vi "Modbus FVIR Boolean Decode.vi"(8 "error in":errorcluster, 10 "Input Registers":u16[](array[numeric]), 11 "PLC Data":T1) -> (0 "error out":errorcluster, 3 "PLC Data Out":T1)   [LabVIEW 2020, in "Modbus.lvlib"]
uses:
  Modbus.lvlib
  Modbus PLC Data All.ctl
  Modbus FVIR Control.ctl
  Modbus LDO Control.ctl
  WritingDataFile/Data to Save.ctl
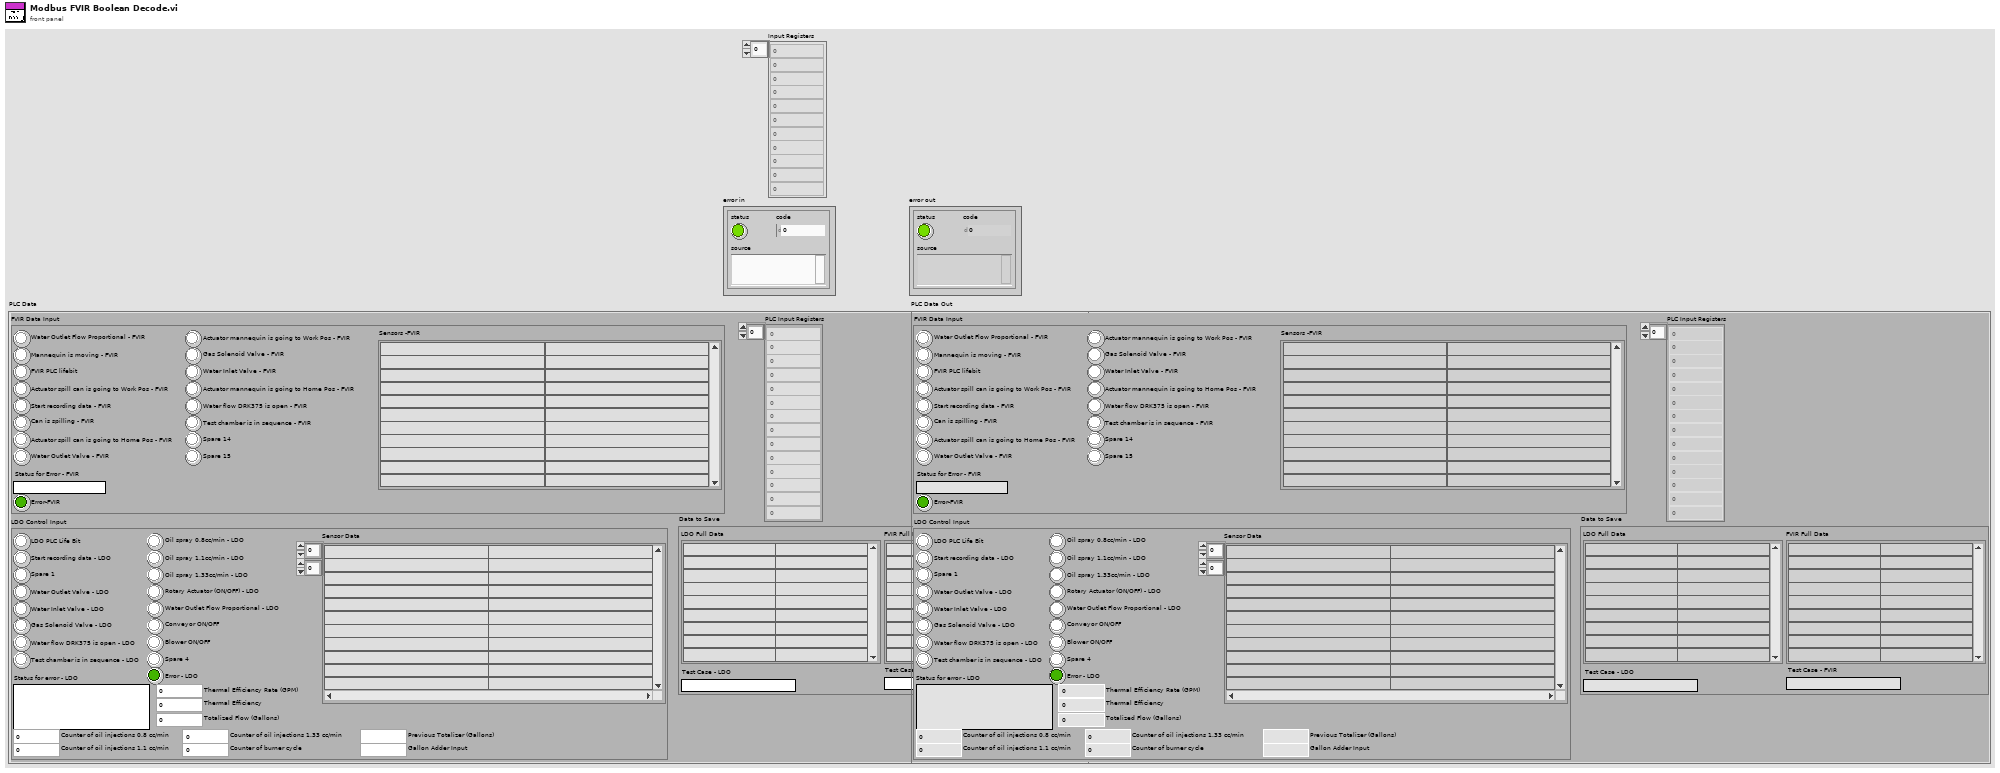
[diagram p1: front panel]
types:
  T1 = typedef "Modbus PLC Data All.ctl" = cluster{"FVIR Data Input":T2, "LDO Control Input":T3, "PLC Input Registers":i16[], "Data to Save":T4}
  T2 = typedef "Modbus FVIR Control.ctl" = cluster{"Spare 15":bool, "Spare 14":bool, "Actuator mannequin is going to Work Pos - FVIR":bool, "Actuator mannequin is going to Home Pos - FVIR":bool, "Test chamber is in sequence - FVIR ":bool, "Water flow DRK375 is open - FVIR":bool, "Gas Solenoid Valve - FVIR":bool, "Water Inlet Valve - FVIR":bool, "Water Outlet Flow Proportional - FVIR":bool, "Start recording data - FVIR":bool, "Actuator spill can is going to Work Pos - FVIR":bool, "Actuator spill can is going to Home Pos - FVIR":bool, "Water Outlet Valve - FVIR":bool, "Can is spilling - FVIR":bool, "Mannequin is moving - FVIR":bool, "FVIR PLC lifebit":bool, "Status for Error - FVIR":string, "Error-FVIR":bool, "Sensors -FVIR":string[][]}
  T3 = typedef "Modbus LDO Control.ctl" = cluster{"LDO PLC Life Bit":bool, "Start recording data - LDO":bool, "Spare 1":bool, "Water Outlet Valve - LDO":bool, "Water Inlet Valve - LDO":bool, "Gas Solenoid Valve - LDO":bool, "Water flow DRK375 is open - LDO":bool, "Test chamber is in sequence - LDO":bool, "Oil spray 0.8cc/min - LDO":bool, "Oil spray 1.1cc/min - LDO":bool, "Oil spray 1.33cc/min - LDO":bool, "Rotary Actuator (ON/OFF) - LDO":bool, "Water Outlet Flow Proportional - LDO":bool, "Conveyor ON/OFF":bool, "Blower ON/OFF":bool, "Spare 4":bool, "Status for error - LDO":string, "Error - LDO":bool, "Sensor Data":string[][], "Thermal Efficiency Rate (GPM)":dbl, "Thermal Efficiency":dbl, "Totalized Flow (Gallons)":dbl, "Counter of oil injections 1.33 cc/min":u16, "Counter of burner cycle":u16, "Counter of oil injections 1.1 cc/min":u16, "Counter of oil injections 0.8 cc/min":u16, "Previous Totalizer (Gallons)":dbl, "Gallon Adder Input":dbl}
  T4 = typedef "Data to Save.ctl" = cluster{"LDO Full Data":string[][], "FVIR Full Data":string[][], "Test Case - FVIR":string, "Test Case - LDO":string}
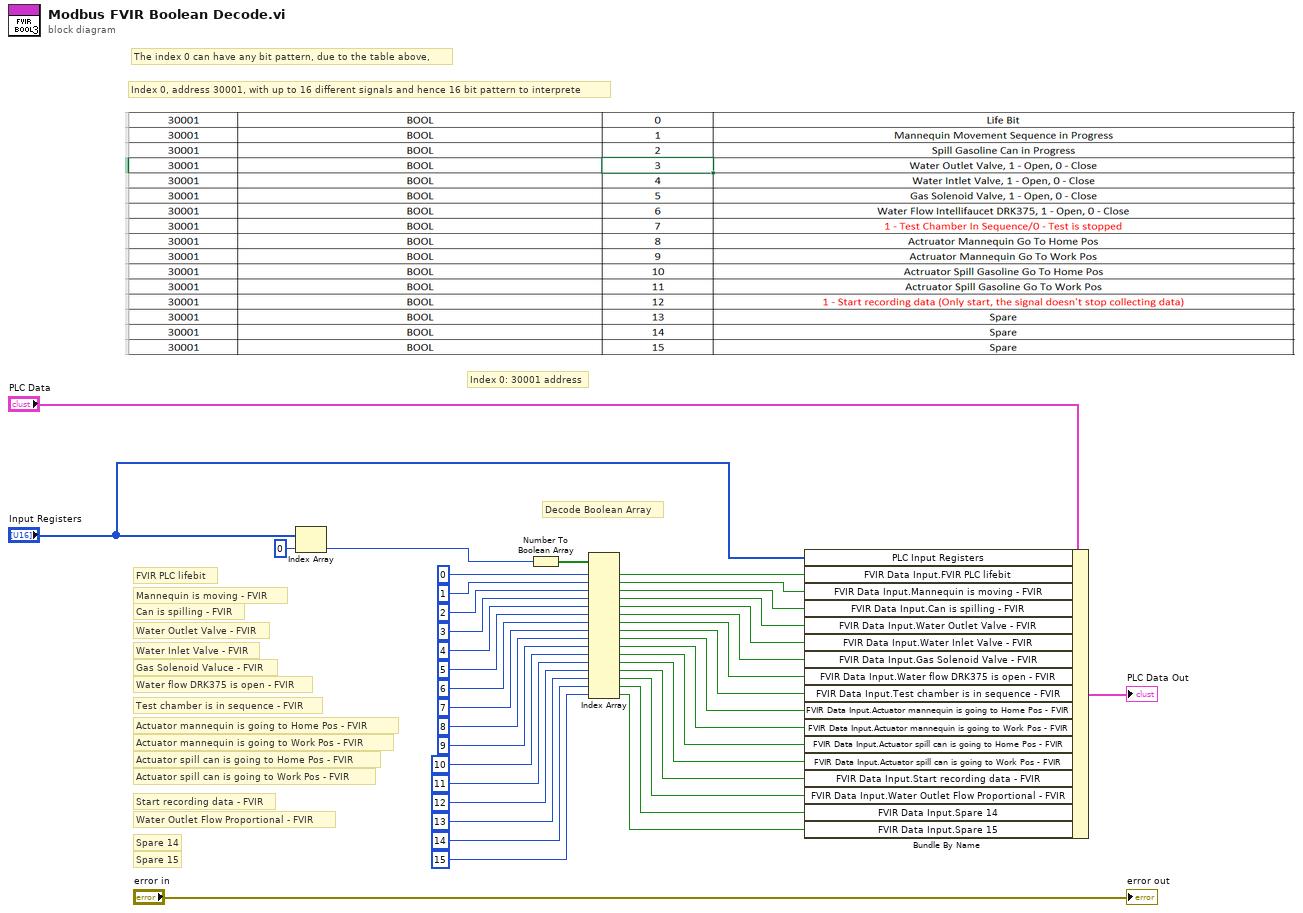
[diagram p0: block diagram]
diagram:
  # "Index 0: 30001 address"
  # "Decode Boolean Array"
  # "Spare 15"
  # "Spare 14"
  # "Water Outlet Flow Proportional - FVIR"
  # "Start recording data - FVIR"
  # "Actuator spill can is going to Work Pos - FVIR"
  # "Actuator spill can is going to Home Pos - FVIR"
  # "Actuator mannequin is going to Work Pos - FVIR"
  # "Actuator mannequin is going to Home Pos - FVIR"
  # "Test chamber is in sequence - FVIR"
  # "Water flow DRK375 is open - FVIR"
  # "Gas Solenoid Valuce - FVIR"
  # "Water Inlet Valve - FVIR"
  # "Water Outlet Valve - FVIR"
  # "Can is spilling - FVIR"
  # "Mannequin is moving - FVIR"
  # "FVIR PLC lifebit"
  # "Index 0, address 30001, with up to 16 different signals and hence 16 bit pattern to interprete"
  # "The index 0 can have any bit pattern, due to the table above,"
  n1 = Index Array(array="Input Registers", index=0) -> (element=w5:u16)
  n2 = Number To Boolean Array(number=w5) -> (Boolean array=w39:bool[])
  n3 = Index Array(array=w39, index #1=0 ("index"), index #2=1 ("index"), index #3=2 ("index"), index #4=3 ("index"), index #5=4 ("index"), index #6=5 ("index"), index #7=6 ("index"), index #8=7 ("index"), index #9=8 ("index"), index #10=9 ("index"), index #11=10 ("index"), index #12=11 ("index"), index #13=12 ("index"), index #14=13 ("index"), index #15=14 ("index"), index #16=15 ("index")) -> (element #1=w22:bool, element #2=w21:bool, element #3=w20:bool, element #4=w19:bool, element #5=w18:bool, element #6=w17:bool, element #7=w16:bool, element #8=w15:bool, element #9=w14:bool, element #10=w13:bool, element #11=w12:bool, element #12=w11:bool, element #13=w10:bool, element #14=w9:bool, element #15=w8:bool, element #16=w7:bool)
  n4 = Bundle By Name(cluster="PLC Data", "PLC Input Registers"="Input Registers", "FVIR Data Input.FVIR PLC lifebit"=w22, "FVIR Data Input.Mannequin is moving - FVIR"=w21, "FVIR Data Input.Can is spilling - FVIR"=w20, "FVIR Data Input.Water Outlet Valve - FVIR"=w19, "FVIR Data Input.Water Inlet Valve - FVIR"=w18, "FVIR Data Input.Gas Solenoid Valve - FVIR"=w17, "FVIR Data Input.Water flow DRK375 is open - FVIR"=w16, "FVIR Data Input.Test chamber is in sequence - FVIR"=w15, "FVIR Data Input.Actuator mannequin is going to Home Pos - FVIR"=w14, "FVIR Data Input.Actuator mannequin is going to Work Pos - FVIR"=w13, "FVIR Data Input.Actuator spill can is going to Home Pos - FVIR"=w12, "FVIR Data Input.Actuator spill can is going to Work Pos - FVIR"=w11, "FVIR Data Input.Start recording data - FVIR"=w10, "FVIR Data Input.Water Outlet Flow Proportional - FVIR"=w9, "FVIR Data Input.Spare 14"=w8, "FVIR Data Input.Spare 15"=w7) -> (→"PLC Data Out":T1)
  "error out" <- "error in"
